vi "ObtenerInformacionProducto.vi"(8 "error in (no error)":errorcluster, 11 "PRODUCTO":string) -> (0 "error out":errorcluster, 2 "Sucess?":bool, 3 "Informacion producto":T1)   [LabVIEW 2020, in "DataBaseSQLlite.lvlib"]
uses:
  DataBaseSQLlite.lvlib
  ProductInvenmtarytyppedef.ctl
  <vilib>/drjdpowell/SQLite Library/SQL Connection/Open (path).vi
  <vilib>/drjdpowell/SQLite Library/SQL Connection/Open (string).vi
  <vilib>/AdvancedString/Path To Command Line String.vi
  <vilib>/drjdpowell/SQLite Library/SQL Connection/Execute SQL (Single Integer).vi
  <vilib>/drjdpowell/SQLite Library/SQL Connection/Connection.lvclass
  <vilib>/drjdpowell/SQLite Library/SQLite.lvlib
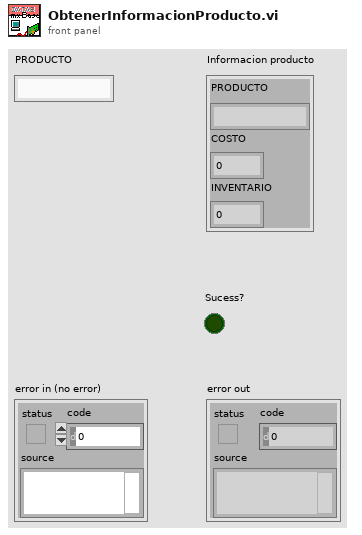
[diagram p1: front panel]
types:
  T1 = cluster{"PRODUCTO":string, "COSTO":dbl, "INVENTARIO":i64}
  T2 = typedef "ProductInvenmtarytyppedef.ctl" = cluster{"PRODUCTO":string, "COSTO":dbl, "INVENTARIO":dbl}
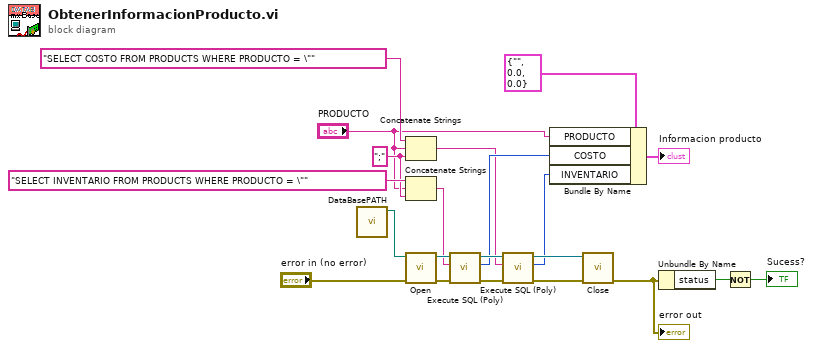
[diagram p0: block diagram]
diagram:
  w6 = ";"
  n1 = call "DataBasePATH.vi"() -> ("DataBase path"=w19:path)  [unwired: 11 in]
  n2 = Concatenate Strings("SELECT COSTO FROM PRODUCTS WHERE PRODUCTO = \"", "PRODUCTO", w6) -> (w1:string)
  n3 = Concatenate Strings("SELECT INVENTARIO FROM PRODUCTS WHERE PRODUCTO = \"", "PRODUCTO", w6) -> (w7:string)
  n4 = call-poly <vilib>:"Open.vi"("error in (no error)"="error in (no error)", "db file"=w19) -> ("error out"=w16:errorcluster, "SQLite Connection"=w17:refnum<class "Connection.lvclass">)  [unwired: 8 in]
  n5 = call-poly <vilib>:"Execute SQL (Poly).vi"("error in (no error)"=w16, "SQL"=w7, "SQLite Connection in"=w17) -> ("error out"=w14:errorcluster, "Result"=w3:i64, "SQLite Connection"=w15:refnum<class "Connection.lvclass">)  [unwired: 6 in]
  n6 = call-poly <vilib>:"Execute SQL (Poly).vi"("error in (no error)"=w14, "SQL"=w1, "SQLite Connection in"=w15) -> ("error out"=w12:errorcluster, "Result"=w2:i64, "SQLite Connection"=w13:refnum<class "Connection.lvclass">)  [unwired: 6 in]
  n7 = Bundle By Name(cluster=T2 {"PRODUCTO"="", "COSTO"=0.0, "INVENTARIO"=0.0} ("Cluster"), "PRODUCTO"="PRODUCTO", "COSTO"=w3, "INVENTARIO"=w2) -> (→"Informacion producto":T2)
  n8 = call-dynamic "Close.vi"("error in (no error)"=w12, "SQLite Connection in"=w13) -> ("error out"=w11:errorcluster)  [unwired: 9 in]
  "error out" <- w11
  n9 = Unbundle By Name(w11) -> ("status"=w10:bool)
  n10 = Not(x=w10) -> (.not. x?=→"Sucess?":bool)
